vi "Handle Command.vi"(8 "error in":errorcluster, 10 "Change Laser Voffset in":refnum<class "Change Laser Voffset.lvclass">, 11 "Object In":refnum<class>) -> (0 "error out":errorcluster, 1 "Command Successful?":bool, 2 "Change Laser Voffset out":refnum<class "Change Laser Voffset.lvclass">, 3 "Object Out":refnum<class>)   [LabVIEW 2014, in "ePAS Library.lvlib" / "Change Laser Voffset.lvclass"]
doc: "Abstract method for accomplishing the execution of a command directed to an instrument object on the wire."
uses:
  Change Laser Voffset.lvclass
  Instrument/ePAS.lvclass
  Instrument/ePAS.lvclass/ePAS.ctl
  reusable/Instrument/Instrument.lvclass/Instrument.ctl
  Change Laser Voffset.lvclass/Change Laser Voffset.ctl
  Instrument/Accessors/Read FPGA Session.vi
  reusable/Instrument/Read Log Session.vi
  <vilib>/Utility/error.llb/Error Cluster From Error Code.vi
  <vilib>/rvi/errors/niLvFpgaAdjustHostInterfaceError.vi
  <userlib>/_Session Fwk/Session - Root.lvclass
  <vilib>/rvi/interface/nirviReadWriteControl/nirviReadWriteControl.xnode
  FPGA/R FPGA Ref.ctl
  FPGA Bitfiles/FPGAServerV2.lvbitx
  FPGA/Session/Exscalabar FPGA.lvclass
  ePAS Library.lvlib
  reusable/Session APIs/Session Log/System Log.lvclass
  NiFpgaLv.dll
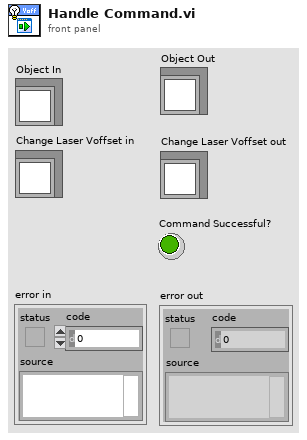
[diagram p1: front panel]
types:
  T1 = typedef "Session - Root.lvclass/Session Handle.ctl" = refnum<data-value>
  T2 = typedef "ePAS Library.lvlib/R FPGA Ref.ctl" = refnum<k20>
  T3 = cluster{"f0":fxp<+,32,0>, "Scale":fxp<+,32,0>, "Offset":i16, "Mod":enum8{"Sine", "Square"}}
  T4 = cluster{"f0":fxp<+,32,0>, "Scale":fxp<+,32,0>, "Offset":i16, "Mod":enum8{"Sine", "Square"}}[]
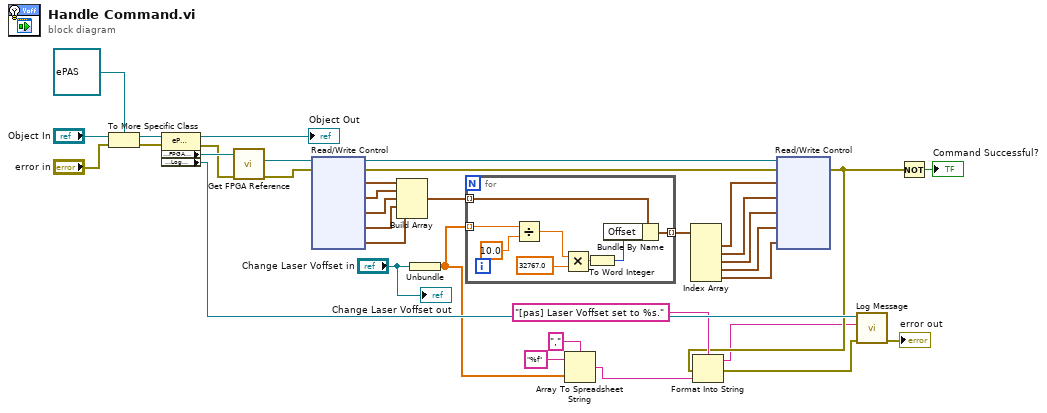
[diagram p0: block diagram]
diagram:
  n1 = To More Specific Class(target class=refnum<class "ePAS.lvclass"> refnum ("ePAS"), reference="Object In", error in="error in") -> (specific class reference=w14:refnum<class "ePAS.lvclass">, error out=w9:errorcluster)
  n2 = property class="ePAS"(reference=w14, error in=w9) -> (reference out=→"Object Out":refnum<class "ePAS.lvclass">, error out=w10:errorcluster, "Accessors:FPGA Session"=w13:T1, "Accessors:Log Session"=w12:T1)
  n3 = call "Get FPGA Reference.vi"("error in"=w10, "Session In"=w13) -> ("error out"=w18:errorcluster, "Ex FPGA Ref"=w34:T2)  [unwired: 7 in, 1 out]
  n4 = xnode "Read/Write Control"("FPGA VI Reference In"=w34, "error in"=w18) -> ("FPGA VI Reference Out"=w27:T2, "error out"=w26:errorcluster, "Cell 1"=w33:T3, "Cell 2"=w32:T3, "Cell 3"=w31:T3, "Cell 4"=w30:T3, "Cell 5"=w29:T3)
  n5 = Build Array(w33, w32, w31, w30, w29) -> (w28:T4)
  n6 = Unbundle("Change Laser Voffset in") -> (w8:dbl[])
  n7 = for {
    tunnel: w28 -> [w44] mode=indexing
    tunnel: w8 -> [w43] mode=indexing
    tunnel: [w42] -> w25 mode=indexing
    n8 = Divide(x=w43, y=10.0) -> (x/y=w40:dbl)
    n9 = Multiply(x=w40, y=32767.0 ("Offset")) -> (x*y=w39:dbl)
    n10 = To Word Integer(number=w39) -> (16bit integer=w38:i16)
    n11 = Bundle By Name(cluster=w44, "Offset"=w38) -> (w42:T3)
  }
  n12 = Array To Spreadsheet String(delimiter (Tab)=",", array=w8, 3:"%f" ("format string")) -> (spreadsheet string=w4:string)
  n13 = Index Array(array=w25) -> (element #1=w24:T3, element #2=w23:T3, element #3=w22:T3, element #4=w21:T3, element #5=w20:T3)  [unwired: 5 in]
  n14 = xnode "Read/Write Control"("FPGA VI Reference In"=w27, "error in"=w26, "Cell 1"=w24, "Cell 2"=w23, "Cell 3"=w22, "Cell 4"=w21, "Cell 5"=w20) -> ("error out"=w3:errorcluster)  [unwired: 1 out]
  n15 = Format Into String(format string="[pas] Laser Voffset set to %s.", error in=w3, w4) -> (resulting string=w1:string, error out=w2:errorcluster)  [unwired: 1 in]
  n16 = call "Log Message.vi"("error in"=w2, "MSG In"=w1, "session in"=w12) -> ("error out"=→"error out":errorcluster)  [unwired: 7 in, 1 out]
  n17 = Not(x=w3) -> (.not. x?=→"Command Successful?":bool)
  "Change Laser Voffset out" <- "Change Laser Voffset in"
